vi "Read Axis origin relative position.vi"(8 "error in (no error)":errorcluster, 11 "Temp params in":refnum<class "CV-Temperature.lvclass">) -> (0 "error out":errorcluster, 2 "Axis origin relative position":dbl=0.5, 3 "Temp params out":refnum<class "CV-Temperature.lvclass">)   [LabVIEW 2013, in "CameraVision.lvlib" / "CV-Temperature.lvclass"]
uses:
  CV-Temperature.lvclass
  CV-Temperature.lvclass/CV-Temperature.ctl
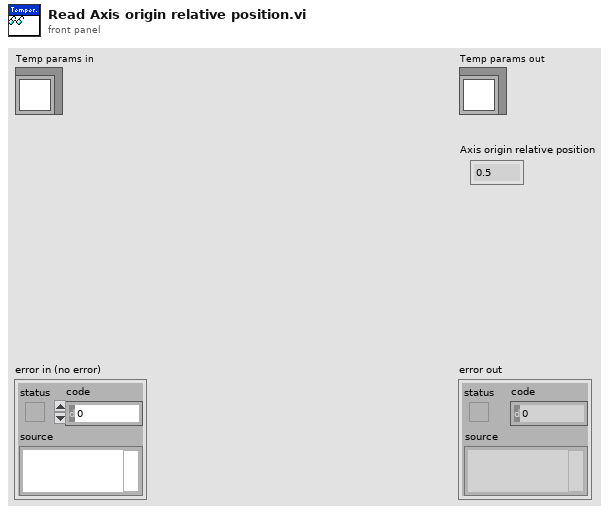
[diagram p1: front panel]
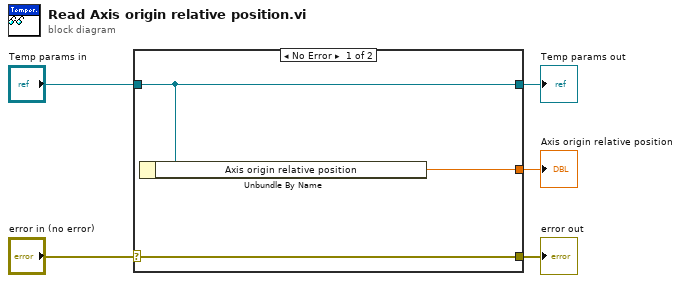
[diagram p0: block diagram]
diagram:
  n1 = case shown="No Error" "error in (no error)" {
    selector: "error in (no error)" -> [w8 w9]
    tunnel: [w8 w9] -> w4
    tunnel: [w7 w10] -> w2
    tunnel: "Temp params in" -> [w7 w10]
    tunnel: [w6 _] -> w1
    frame No Error {
      n2 = Unbundle By Name(w7) -> ("Axis origin relative position"=w6:dbl)
    }
    frame Error {
    }
  }
  "error out" <- w4
  "Temp params out" <- w2
  "Axis origin relative position" <- w1
